vi "Do.vi"(8 "error in (no error)":errorcluster, 10 "Actor in":refnum<class "Actor.lvclass">, 11 "Request Update from Process Msg":refnum<class "Request Update from Process Msg.lvclass">) -> (0 "error out":errorcluster, 2 "Actor out":refnum<class "Actor.lvclass">)   [LabVIEW 2025, in "Process States.lvlib" / "Request Update from Process Msg.lvclass"]
doc: "This VI delivers the message to the actor by calling the appropriate method(s) on the actor."
uses:
  Request Update from Process Msg.lvclass
  <vilib>/ActorFramework/Actor/Actor.lvclass
  Idle/Idle.lvclass
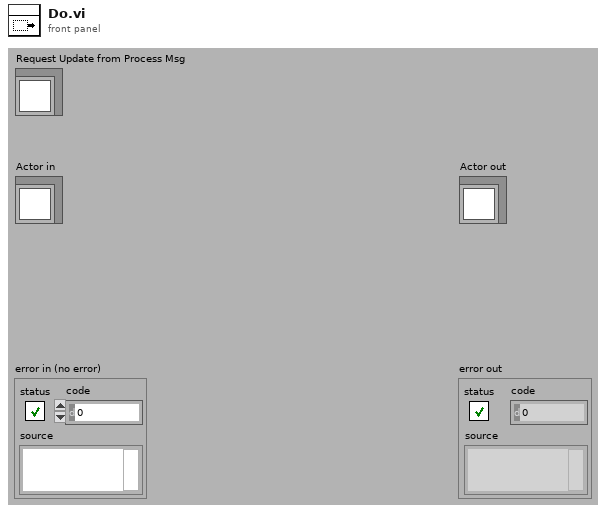
[diagram p1: front panel]
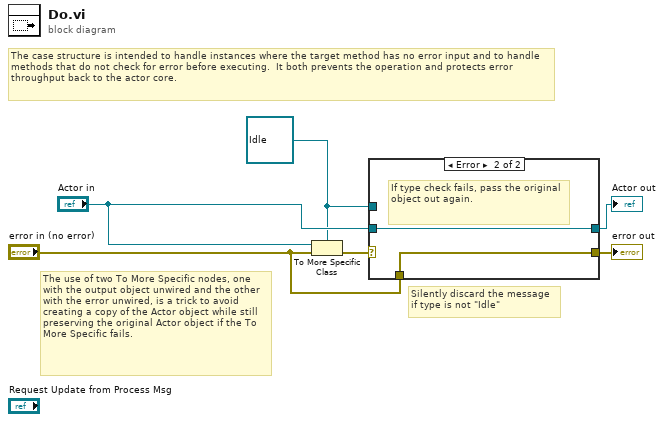
[diagram p0: block diagram]
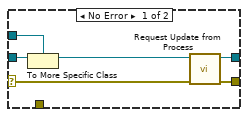
[diagram p2: hidden frame]
diagram:
  w2 = refnum<class "Idle.lvclass"> refnum ("Actor in")
  # "Silently discard the message\nif type is not \"Idle\""
  # "The use of two To More Specific nodes, one with the output object unwired and the other with the error unwired, is a trick to avoid creating a copy of the Actor object while still preserving the original Actor object if the To More Specific fails."
  # "The case structure is intended to handle instances where the target method has no error input and to handle methods that do not check for error before executing.  It both prevents the operation and protects error throughput back to the actor core."
  n1 = To More Specific Class(target class=w2, reference="Actor in", error in="error in (no error)") -> (error out=w6:errorcluster)  [unwired: 1 out]
  n2 = case shown="Error" w6 {
    selector: w6 -> [w10 _]
    tunnel: [w12 w13] -> w5
    tunnel: [w11 w14] -> w4
    tunnel: "Actor in" -> [w9 w14]
    tunnel: w2 -> [w8 _]
    tunnel: "error in (no error)" -> [_ w13]
    frame No Error {
      n3 = To More Specific Class(target class=w8, reference=w9) -> (specific class reference=w7:refnum<class "Idle.lvclass">)  [unwired: 1 in, 1 out]
      n4 = call "Request Update from Process.vi"("error in (no error)"=w10, "Ilde in"=w7) -> ("error out"=w12:errorcluster, "Ilde out"=w11:refnum<class "Idle.lvclass">)  [unwired: 8 in]
    }
    frame Error {
      # "If type check fails, pass the original object out again."
    }
  }
  "error out" <- w5
  "Actor out" <- w4
